vi "WHILE.vi"() -> ()   [LabVIEW 2020]
uses:
  <vilib>/numeric/Random Number (Range) DBL.vi
panel:
  out "DATOS OBTENIDOS":string[][](array[string])
  out "Waveform Chart":dynamicdata(graph)
  out "RANGO":bool
  out "N° LÍMITE MÁXIMO":dbl
  out "ON/OFF":bool
  out "SEÑAL ANALÓGICA SIN FILTRAR":dbl
  in  "PARO DEL CILCLO":bool
  # "DIEGO JÁUREGUI ONTIVEROS 3MM4"
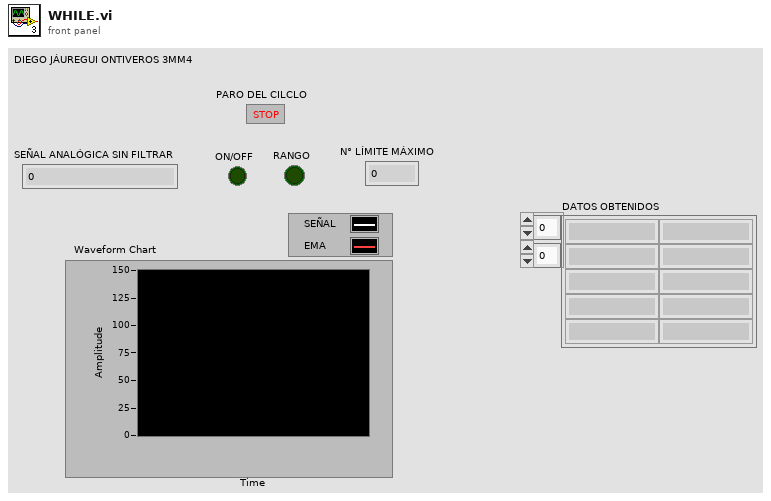
[diagram p1: front panel]
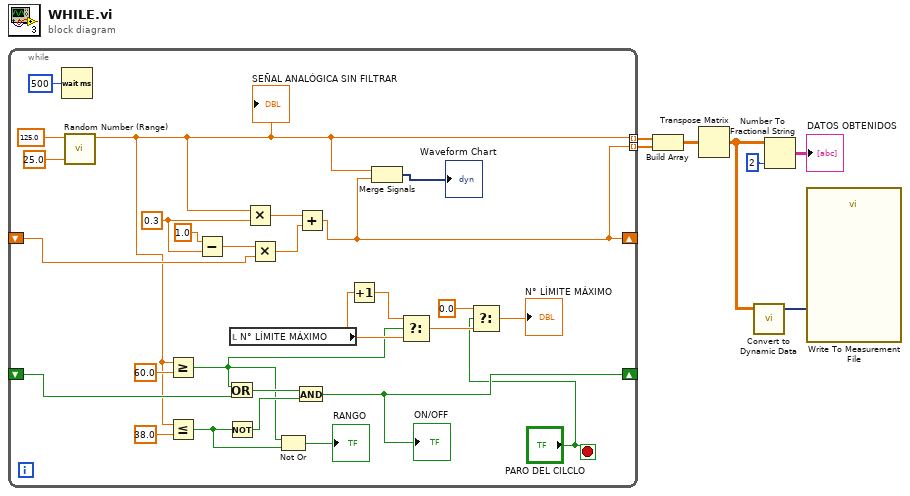
[diagram p0: block diagram]
diagram:
  n1 = while {
    shift-right: [w8] -> _
    shift-left: _ -> [w18]
    shift-right: [w16] -> _
    shift-left: _ -> [w17]
    tunnel: [w9] -> w7 mode=indexing
    tunnel: [w8] -> w6 mode=indexing
    stop <- "PARO DEL CILCLO" stop-if-true
    w31 = 0.3
    n2 = Wait (ms)(milliseconds to wait=u32 500) -> ()  [unwired: 1 out]
    n3 = call-poly <vilib>:"Random Number (Range).vi"("lower bound (0)"=25.0, "upper bound (100)"=125.0) -> ("number"=w9:dbl)  [unwired: 9 in]
    "SEÑAL ANALÓGICA SIN FILTRAR" <- w9
    n4 = Greater Or Equal?(x=w9, y=60.0) -> (x >= y?=w20:bool)
    n5 = Less Or Equal?(x=w9, y=38.0) -> (x <= y?=w19:bool)
    n6 = Subtract(x=1.0, y=w31) -> (x-y=w29:dbl)
    n7 = Or(x=w20, y=w17) -> (x .or. y?=w26:bool)
    n8 = Not(x=w19) -> (.not. x?=w27:bool)
    n9 = local read "N° LÍMITE MÁXIMO"() -> (w22:dbl)
    n10 = Multiply(x=w9, y=w31) -> (x*y=w28:dbl)
    n11 = Multiply(x=w29, y=w18) -> (x*y=w30:dbl)
    n12 = Not Or(1:w19, 2:w20) -> (0:→"RANGO":bool)
    n13 = And(x=w26, y=w27) -> (x .and. y?=w16:bool)
    "ON/OFF" <- w16
    n14 = Add(x=w28, y=w30) -> (x+y=w8:dbl)
    n15 = Increment(x=w22) -> (x+1=w23:dbl)
    n16 = Merge Signals(w9, w8) -> (→"Waveform Chart":dynamicdata)
    n17 = Select(t=w23, s=w20, f=w22) -> (s? t:f=w13:dbl)
    n18 = Select(t=0.0, s="PARO DEL CILCLO", f=w13) -> (s? t:f=→"N° LÍMITE MÁXIMO":dbl)
  }
  n19 = Build Array(w7, w6) -> (w1:dbl[][])
  n20 = Transpose Matrix(1:w1) -> (0:w4:dbl[][])
  n21 = call "Convert to Dynamic Data"("2D Array"=w4) -> ("Dynamic Data Type"=w3:dynamicdata)  [unwired: 3 in]
  n22 = Number To Fractional String(number=w4, precision (6)=i16 2) -> (F-format string=→"DATOS OBTENIDOS":string[][])  [unwired: 2 in]
  n23 = call "Write To Measurement File"("Signals"=w3) -> ()  [unwired: 16 in, 3 out]
